vi "PH_AxisGUI_BaseClass.PC Clear Error.vi"(0 "i ref in":refnum<vi>, 2 "Axis":i32=-1, 5 "error in":errorcluster) -> (14 "i ref out":refnum<vi>, 19 "error out":errorcluster)   [LabVIEW 2014, in "PH_AxisGUI_BaseClass.lvlib"]
doc: "This VI acts on an axis."
uses:
  PH_AxisGUI_BaseClass.lvlib
  PH_Stepmotor_BaseClass/PH_Stepmotor_BaseClass.lvlib
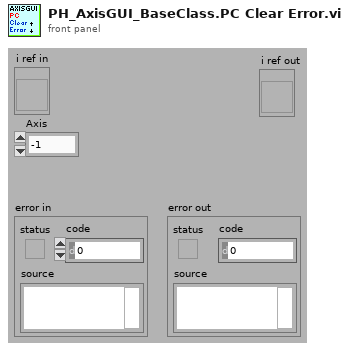
[diagram p1: front panel]
types:
  T1 = typedef "PH_Stepmotor_BaseClass.lvlib/PH_Stepmotor_BaseClass.Axis Address.ctl" = cluster{"Instance":string, "Motor Nr":i32}
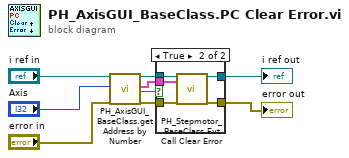
[diagram p0: block diagram]
diagram:
  n1 = call "PH_AxisGUI_BaseClass.get Address by Number.vi"("VI in"="i ref in", "Axis"="Axis", "error in (no error)"="error in") -> ("VI out"=w4:refnum<vi>, "Address"=w2:T1, "Axis exists and is not moving?"=w1:bool, "error out"=w3:errorcluster)  [unwired: 12 in, 1 out]
  n2 = case "Axis moving or no motion instance?" shown="True" w1 {
    tunnel: [w11 w12] -> w7
    tunnel: [w10 w13] -> w6
    tunnel: w4 -> [w11 w16]
    tunnel: w3 -> [w10 w15]
    tunnel: w2 -> [_ w14]
    frame False {
    }
    frame True {
      n3 = call "PH_Stepmotor_BaseClass.Evt Call Clear Error.vi"("i ref in"=w16, "Address"=w14, "error in"=w15) -> ("i ref out"=w12:refnum<vi>, "error out"=w13:errorcluster)  [unwired: 15 in]
    }
  }
  "error out" <- w6
  "i ref out" <- w7
